vi "Read Settings File.vi"(8 "Error In":errorcluster, 11 "Settings Filepath":path) -> (0 "Error Out":errorcluster)   [LabVIEW 2023, in "Error Manager.lvlib" / "Settings.lvclass"]
doc: "This VI reads and parses the Error Manager Settings file (a.k.a. config file or ini file). The setting values are then stored in a LabVIEW object."
uses:
  Settings.lvclass
  Settings.lvclass/Settings.ctl
  Error Manager.lvlib
  <vilib>/Utility/config.llb/NI_LVConfig.lvlib
panel:
  # "Input\nInputs to the VI"
  # "Development\nControls or indicators that are useful for development or testing, but which are not outputs of the VI."
  # "Output\nOutputs of the VI"
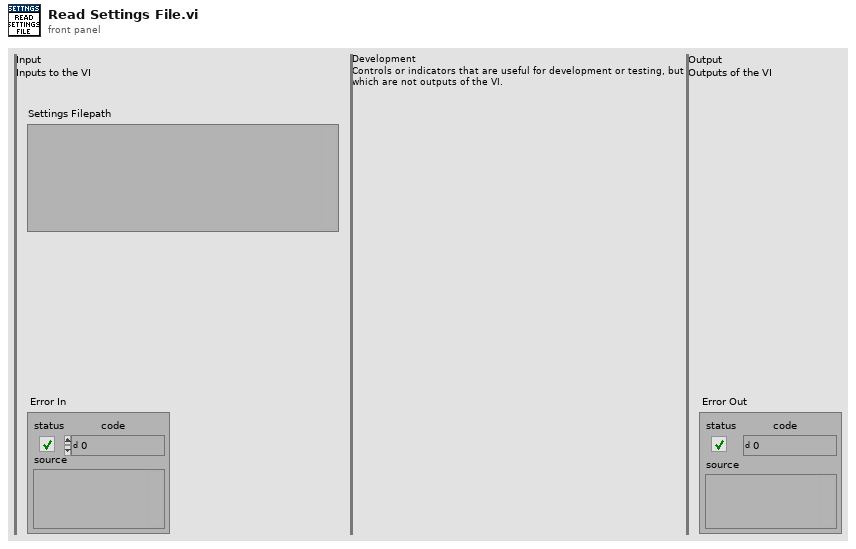
[diagram p1: front panel]
types:
  T1 = typedef "NI_LVConfig.lvlib/Config Data RefNum.ctl" = refnum<k1>
  T2 = typedef "Error Manager.lvlib/Settings.lvclass/Error_Log_Setting (enum).ctl" = enum16{"Log Full Error Details", "Log Error Codes Only", "Do Not Log"}
  T3 = typedef "Error Manager.lvlib/Settings.lvclass/Window_Behaviour (enum).ctl" = enum16{"Default", "Floating", "Modal"}
  T4 = typedef "Error Manager.lvlib/Settings.lvclass/Show_Error_Window_Default (enum).ctl" = enum16{"For All Errors", "For New Errors", "For New Error Codes", "Never"}
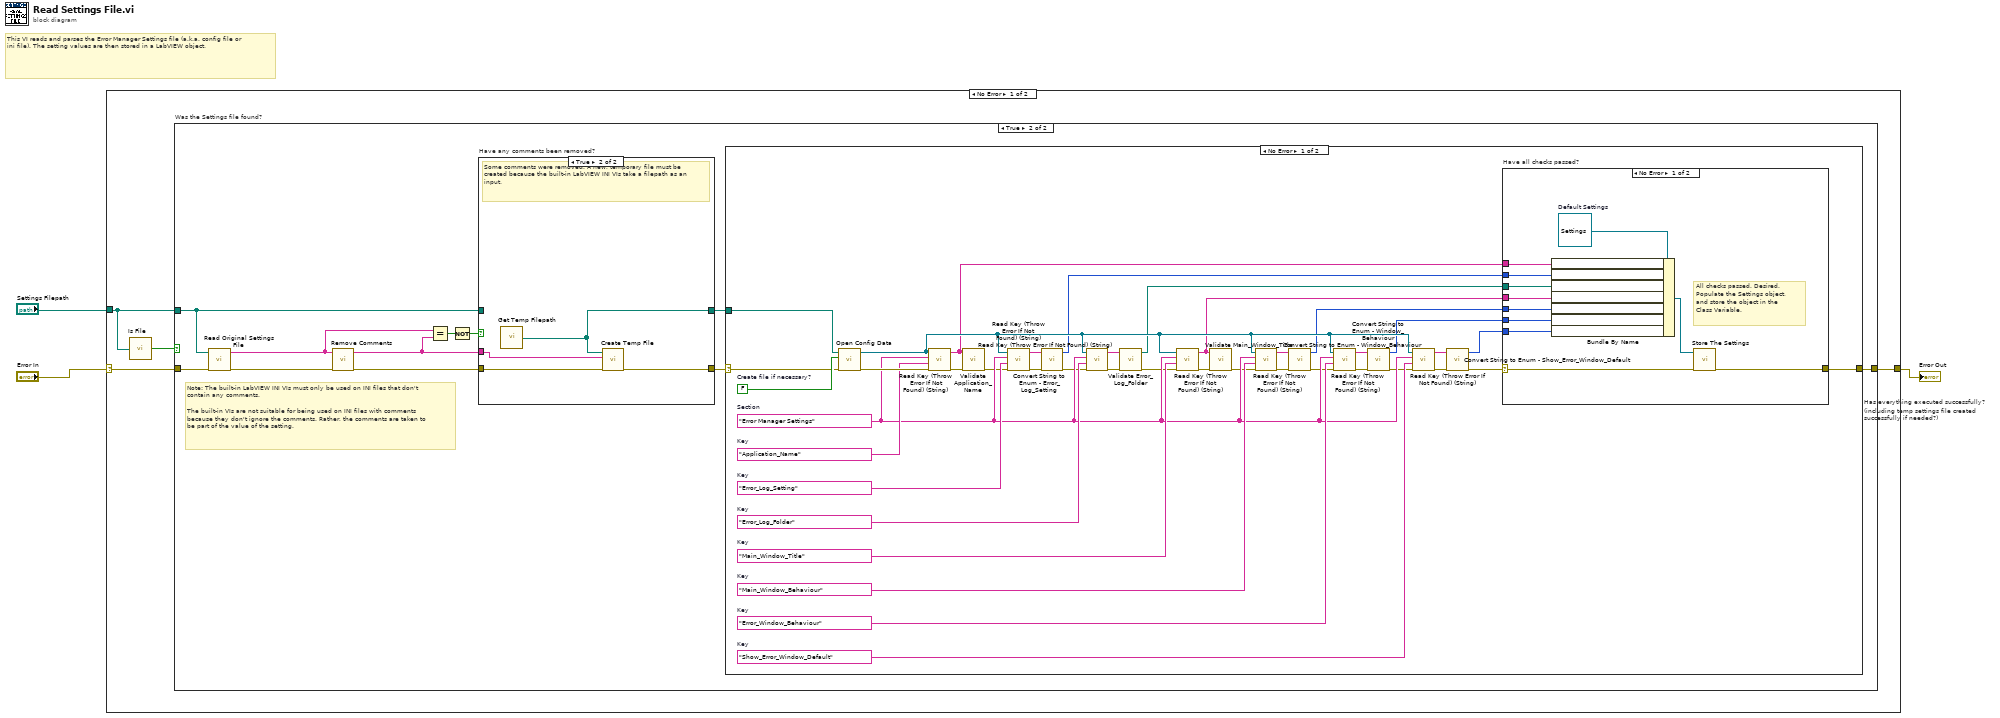
[diagram p0: block diagram]
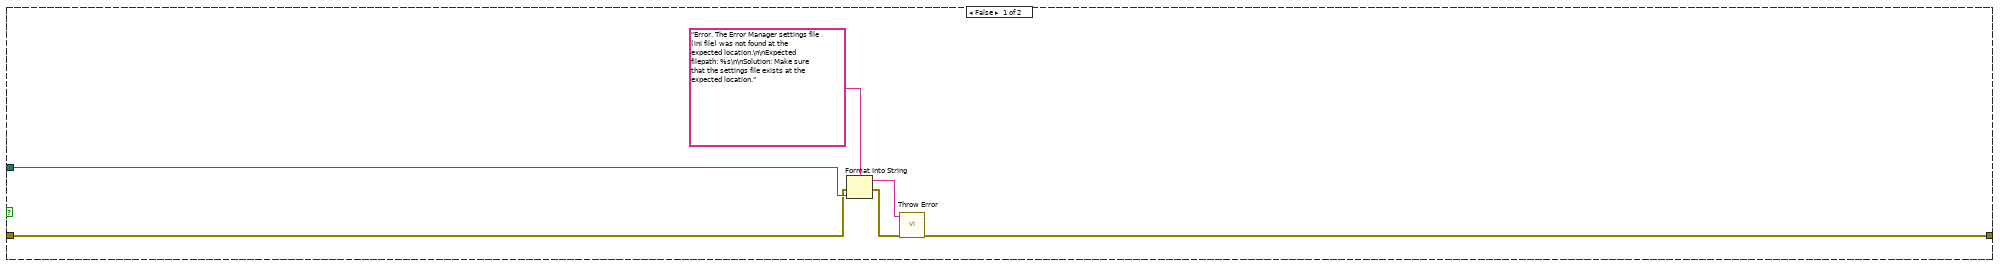
[diagram p2: hidden frame]
diagram:
  # "This VI reads and parses the Error Manager Settings file (a.k.a. config file or ini file). The setting values are then stored in a LabVIEW object."
  n1 = case shown="No Error" "Error In" {
    selector: "Error In" -> [w7 w84]
    tunnel: [w6 w84] -> w2
    tunnel: "Settings Filepath" -> [w4 _]
    frame No Error {
      n2 = call "Is File.vi"(1:w4) -> (0:w5:bool)
      n3 = case "Was the Settings file found?" shown="True" w5 {
        tunnel: w7 -> [w9 w24]
        tunnel: [w13 w22] -> w6
        tunnel: w4 -> [w11 w21]
        frame False {
          n4 = Format Into String(format string="Error. The Error Manager settings file (ini file) was not found at the expected location.\n\nExpected filepath: %s\n\nSolution: Make sure that the settings file exists at the expected location.", error in=w9, w11) -> (resulting string=w8:string, error out=w10:errorcluster)  [unwired: 1 in]
          n5 = call "Throw Error.vi"(8:w10, 11:w8) -> (0:w13:errorcluster)  [unwired: 9 in]
        }
        frame True {
          # "Note: The built-in LabVIEW INI VIs must only be used on INI files that don't contain any comments.\n\nThe built-in VIs are not suitable for being used on INI files with comments because they don't ignore the comments. Rather, the comments are taken to be part of the value of the setting."
          n6 = call "Read Original Settings File.vi"(8:w24, 11:w21) -> (0:w20:errorcluster, 3:w18:string)  [unwired: 8 in]
          n7 = call "Remove Comments.vi"(8:w20, 11:w18) -> (0:w19:errorcluster, 3:w14:string)  [unwired: 8 in]
          n8 = Equal?(x=w18, y=w14) -> (x = y?=w17:bool)
          n9 = Not(x=w17) -> (.not. x?=w16:bool)
          n10 = case "Have any comments been removed?" shown="True" w16 {
            tunnel: [w26 w30] -> w23
            tunnel: w21 -> [w25 _]
            tunnel: w19 -> [w26 w29]
            tunnel: [w25 w28] -> w15
            tunnel: w14 -> [_ w27]
            frame False {
              # "There is no need to create a temp file. The INI VIs can be used to read directly from the original settings file."
              # "The original settings file does not contain any comments."
            }
            frame True {
              # "Some comments were removed. A new, temporary file must be created because the built-in LabVIEW INI VIs take a filepath as an input."
              n11 = call "Get Temp Filepath.vi"() -> (w28:path)
              n12 = call "Create Temp File.vi"(8:w29, 10:w27, 11:w28) -> (0:w30:errorcluster)  [unwired: 8 in]
            }
          }
          n13 = case "Has everything executed successfully? (including temp settings file created successfully if needed?)" shown="No Error" w23 {
            selector: w23 -> [w69 w83]
            tunnel: [w31 w83] -> w22
            tunnel: w15 -> [w68 _]
            frame No Error {
              w57 = "Show_Error_Window_Default"  # Key
              w59 = "Error_Window_Behaviour"  # Key
              w60 = "Main_Window_Behaviour"  # Key
              w62 = "Main_Window_Title"  # Key
              w64 = "Error_Log_Folder"  # Key
              w65 = "Error_Log_Setting"  # Key
              w66 = "Application_Name"  # Key
              w58 = "Error Manager Settings"  # Section
              w70 = FALSE  # Create file if necessary?
              n14 = call <vilib>:"Open Config Data.vi"(8:w69, 10:w70, 11:w68) -> (0:w67:errorcluster, 3:w53:T1)  [unwired: 6 in, 1 out]
              n15 = call "Read Key (Throw Error If Not Found) (String).vi"(8:w67, 9:w66, 10:w58, 11:w53) -> (0:w52:errorcluster, 3:w47:string)  [unwired: 6 in]
              n16 = call "Validate Application_Name.vi"(8:w52, 11:w47) -> (0:w51:errorcluster)  [unwired: 9 in]
              n17 = call "Read Key (Throw Error If Not Found) (String).vi"(8:w51, 9:w65, 10:w58, 11:w53) -> (0:w50:errorcluster, 3:w48:string)  [unwired: 6 in]
              n18 = call "Convert String to Enum - Error_Log_Setting.vi"(8:w50, 11:w48) -> (0:w49:errorcluster, 3:w46:T2)  [unwired: 8 in]
              n19 = call "Read Key (Throw Error If Not Found) (String).vi"(8:w49, 9:w64, 10:w58, 11:w53) -> (0:w63:errorcluster, 3:w33:string)  [unwired: 6 in]
              n20 = call "Validate Error_Log_Folder.vi"(8:w63, 11:w33) -> (0:w34:errorcluster, 3:w32:path)  [unwired: 8 in]
              n21 = call "Read Key (Throw Error If Not Found) (String).vi"(8:w34, 9:w62, 10:w58, 11:w53) -> (0:w61:errorcluster, 3:w38:string)  [unwired: 6 in]
              n22 = call "Validate Main_Window_Title.vi"(8:w61, 11:w38) -> (0:w45:errorcluster)  [unwired: 9 in]
              n23 = call "Read Key (Throw Error If Not Found) (String).vi"(8:w45, 9:w60, 10:w58, 11:w53) -> (0:w56:errorcluster, 3:w43:string)  [unwired: 6 in]
              n24 = call "Convert String to Enum - Window_Behaviour.vi"(8:w56, 11:w43) -> (0:w44:errorcluster, 3:w42:T3)  [unwired: 8 in]
              n25 = call "Read Key (Throw Error If Not Found) (String).vi"(8:w44, 9:w59, 10:w58, 11:w53) -> (0:w55:errorcluster, 3:w40:string)  [unwired: 6 in]
              n26 = call "Convert String to Enum - Window_Behaviour.vi"(8:w55, 11:w40) -> (0:w41:errorcluster, 3:w39:T3)  [unwired: 8 in]
              n27 = call "Read Key (Throw Error If Not Found) (String).vi"(8:w41, 9:w57, 10:w58, 11:w53) -> (0:w54:errorcluster, 3:w36:string)  [unwired: 6 in]
              n28 = call "Convert String to Enum - Show_Error_Window_Default.vi"(8:w54, 11:w36) -> (0:w37:errorcluster, 3:w35:T4)  [unwired: 8 in]
              n29 = case "Have all checks passed?" shown="No Error" w37 {
                selector: w37 -> [w76 w82]
                tunnel: w47 -> [w81 _]
                tunnel: w46 -> [w80 _]
                tunnel: w42 -> [w79 _]
                tunnel: w39 -> [w78 _]
                tunnel: w38 -> [w77 _]
                tunnel: w35 -> [w75 _]
                tunnel: w32 -> [w74 _]
                tunnel: [w73 w82] -> w31
                frame No Error {
                  w71 = refnum<class "Settings.lvclass"> refnum  # Default Settings
                  # "All checks passed. Desired. Populate the Settings object, and store the object in the Class Variable."
                  n30 = Bundle By Name(cluster=w71, w81, w80, w74, w77, w79, w78, w75) -> (w72:refnum<class "Settings.lvclass">)
                  n31 = call "Store The Settings.vi"(8:w76, 11:w72) -> (0:w73:errorcluster)  [unwired: 9 in]
                }
                frame Error {
                  # "One or more checks failed.\n\nThere are one or more invalid settings values."
                }
              }
            }
            frame Error {
            }
          }
        }
      }
    }
    frame Error {
    }
  }
  "Error Out" <- w2
